vi "Get Parent and DMA Type.vi"(8 "error in (no error)":errorcluster, 11 "Node Ptr":T1 format="%.0x") -> (0 "error out":errorcluster, 1 "Input?":bool, 2 "Parent Ref":T1 format="%.0x", 3 "Item Ref out":T1 format="%.0x")   [LabVIEW 2019, in "FPGA Addon System Explorer.lvlib"]
uses:
  FPGA Addon System Explorer.lvlib
  <vilib>/NI VeriStand/Custom Device API/Custom Device Item Ref.ctl
  Addon Shared/SubVIs/Constants.vi
  <vilib>/NI VeriStand/Custom Device API/Custom Device API.lvlib
  Addon Shared/FPGA Addon Shared.lvlib
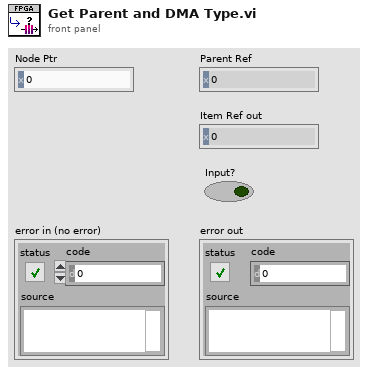
[diagram p1: front panel]
types:
  T1 = typedef "Custom Device API.lvlib/Custom Device Item Ref.ctl" = u64
  T2 = typedef "Custom Device API.lvlib/Custom Device Item Info.ctl" = cluster{"Name":string, "Is Channel":bool, "GUID":string, "Is Waveform":bool}
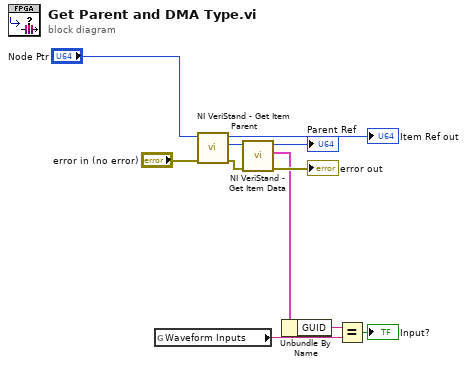
[diagram p0: block diagram]
diagram:
  n1 = global read "Constants.vi" "Waveform Inputs"() -> (w10:string)
  n2 = call <vilib>:"NI VeriStand - Get Item Parent.vi"("error in (no error)"="error in (no error)", "Item Ref in"="Node Ptr") -> ("error out"=w5:errorcluster, "Parent Ref"=w4:T1, "Item Ref out"=→"Item Ref out":T1)  [unwired: 6 in, 1 out]
  n3 = call <vilib>:"NI VeriStand - Get Item Data.vi"("error in (no error)"=w5, "Item Ref in"=w4) -> ("error out"=→"error out":errorcluster, "Item Info"=w6:T2, "Item Ref out"=→"Parent Ref":T1)  [unwired: 7 out]
  n4 = Unbundle By Name(w6) -> ("GUID"=w9:string)
  n5 = Equal?(x=w9, y=w10) -> (x = y?=→"Input?":bool)
